vi "DFD FXP to I16 (scalar).vi"(7 "quantization settings":T1={"source"=0, "wl"=16, "iwl"=1, "overflow mode"=enum."Wrap", "rounding mode"=enum."Truncation", "signed?"=TRUE} {"source" items=["Coefficients a/k"=0, "Coefficients b/v"=7, "Input"=1, "Output"=2, "Multiplicand"=3, "Product"=4, "Sum"=5, "Delay"=6]}, 8 "error in (no error)":errorcluster, 11 "FXP value":dbl) -> (0 "error out":errorcluster, 3 "I16":i16)   [LabVIEW 2017, in "NI_DigFilterLicensed.lvlib"]
doc: "Converts fixed-point numbers to integers. You must manually select the polymorphic instance you want to use."
uses:
  <vilib>/addons/Digital Filter Design/NI_DigFilterLicensed.lvlib
  <vilib>/addons/Digital Filter Design/_Objects.llb/DFD Quantization Settings.ctl
  <vilib>/addons/Digital Filter Design/_Objects.llb/DFD Quantization Sources.ctl
  <vilib>/addons/Digital Filter Design/FXPLib.llb/dfd_FXP Casting (scaler).vi
  <vilib>/addons/Digital Filter Design/NI_DigFilter_FXP.lvlib
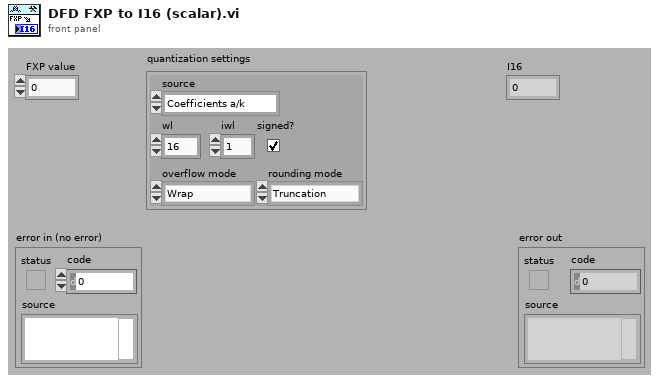
[diagram p1: front panel]
types:
  T1 = typedef "NI_DigFilterLicensed.lvlib/DFD Quantization Settings.ctl" = cluster{"source":T2, "wl":i16, "iwl":i16, "overflow mode":enum16{"Saturation", "Wrap"}, "rounding mode":enum16{"Nearest", "Truncation"}, "signed?":bool}
  T2 = typedef "NI_DigFilterLicensed.lvlib/DFD Quantization Sources.ctl" = u16
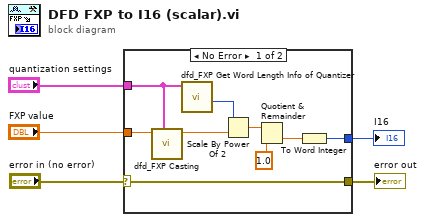
[diagram p0: block diagram]
diagram:
  n1 = case shown="No Error" "error in (no error)" {
    selector: "error in (no error)" -> [w6 w15]
    tunnel: [w12 _] -> w5
    tunnel: "FXP value" -> [w11 _]
    tunnel: "quantization settings" -> [w7 _]
    tunnel: [w6 w15] -> w1
    frame No Error {
      n2 = call-poly <vilib>:"dfd_FXP Casting.vi"("quantization settings"=w7, "value in"=w11) -> ("value out"=w9:dbl)  [unwired: 1 in, 6 out]
      n3 = call <vilib>:"dfd_FXP Get Word Length Info of Quantizer.vi"("quantization settings"=w7) -> ("fwl"=w8:i16)  [unwired: 10 out]
      n4 = Scale By Power Of 2(n=w8, x=w9) -> (x*2^n=w10:dbl)
      n5 = Quotient & Remainder(x=w10, y=1.0) -> (floor(x/y)=w13:dbl)  [unwired: 1 out]
      n6 = To Word Integer(number=w13) -> (16bit integer=w12:i16)
    }
    frame Error {
    }
  }
  "I16" <- w5
  "error out" <- w1
